vi "Load File.vi"(8 "error in (no error)":errorcluster, 11 "error codes file":path) -> (0 "error out":errorcluster, 1 "errors":T2[](array[typedef]), 2 "comment":string, 3 "family":T1, 5 "parsable?":bool)   [LabVIEW 2017, in "Error File Management.lvlib"]
uses:
  Error File Management.lvlib
  Controls/NI Error.ctl
  Controls/NI Family.ctl
  <vilib>/xml/Load XML File.vi
  <vilib>/xml/Close Reference(Node).vi
  <vilib>/xml/NI_XML.lvlib
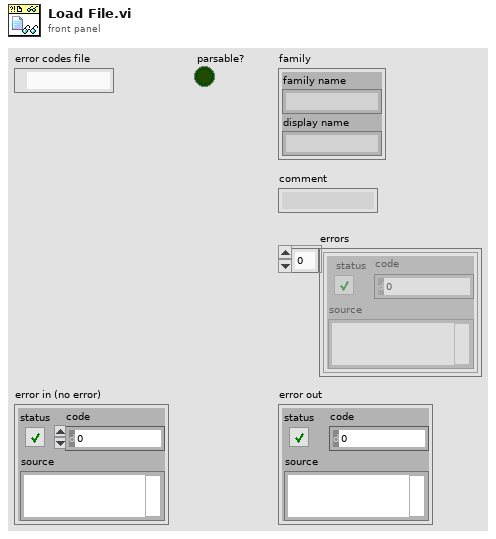
[diagram p1: front panel]
types:
  T1 = typedef "Error File Management.lvlib/NI Family.ctl" = cluster{"family name":string, "display name":string}
  T2 = typedef "Error File Management.lvlib/NI Error.ctl" = errorcluster
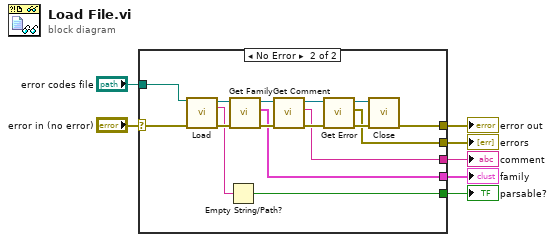
[diagram p0: block diagram]
diagram:
  n1 = case shown="No Error" "error in (no error)" {
    selector: "error in (no error)" -> [w8 w12]
    tunnel: [_ w21] -> w7
    tunnel: [_ w20] -> w6
    tunnel: [_ w19] -> w5
    tunnel: "error codes file" -> [_ w11]
    tunnel: [w8 w13] -> w2
    tunnel: [_ w9] -> w1
    frame Error {
    }
    frame No Error {
      n2 = call-poly <vilib>:"Load.vi"("path to XML document"=w11, "error in (no error)"=w12) -> ("DOM document out"=w14:refnum<k20>, "parse errors"=w10:string, "error out"=w15:errorcluster)  [unwired: 11 in]
      n3 = Empty String/Path?(string/path=w10) -> (empty?=w9:bool)
      n4 = call "Get Family.vi"("error in (no error)"=w15, "DOM document in"=w14) -> ("error out"=w22:errorcluster, "family"=w20:T1, "DOM document out"=w16:refnum<k20>)  [unwired: 7 in]
      n5 = call "Get Comment.vi"("error in (no error)"=w22, "DOM document in"=w16) -> ("error out"=w23:errorcluster, "comment"=w19:string, "DOM document out"=w17:refnum<k20>)  [unwired: 7 in]
      n6 = call "Get Error.vi"("error in (no error)"=w23, "DOM document in"=w17) -> ("error out"=w24:errorcluster, "errors"=w21:T2[], "DOM document out"=w18:refnum<k20>)  [unwired: 7 in]
      n7 = call-poly <vilib>:"Close.vi"("error in (no error)"=w24, "node"=w18) -> ("error out"=w13:errorcluster)  [unwired: 7 in]
    }
  }
  "errors" <- w7
  "family" <- w6
  "comment" <- w5
  "error out" <- w2
  "parsable?" <- w1
